vi "Open Device.vi"(8 "error in (no error)":errorcluster, 11 "Simulated Scope in":refnum<class "Simulated Scope.lvclass">) -> (0 "error out":errorcluster, 3 "Simulated Scope out":refnum<class "Simulated Scope.lvclass">)   [LabVIEW 2020, in "Simulated Scope.lvlib" / "Simulated Scope.lvclass"]
uses:
  Simulated Scope.lvclass
  Simulated Scope.lvclass/Simulated Scope.ctl
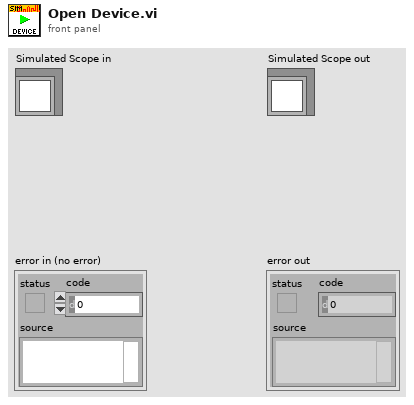
[diagram p1: front panel]
types:
  T1 = typedef "Simulated Scope.lvlib/Simulated Scope.lvclass/Ref Data.ctl" = cluster{"Sim Queue Name":string, "Waveform Queue":refnum<queue>}
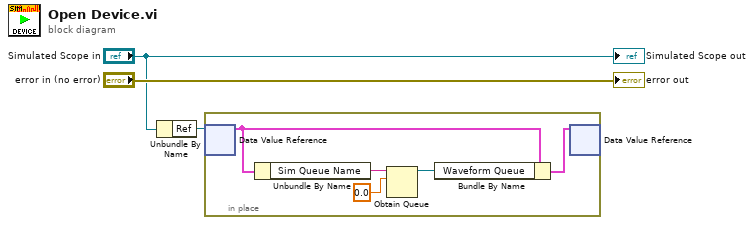
[diagram p0: block diagram]
diagram:
  n1 = Unbundle By Name("Simulated Scope in") -> ("Ref"=w3:refnum<data-value>)
  n2 = in-place {
    n3 = in-place-dvr #1(w3) -> (w6:T1)  [unwired: 1 out]
    n4 = Unbundle By Name(w6) -> ("Sim Queue Name"=w8:string)
    n5 = Obtain Queue(name (unnamed)=w8, element data type=0.0) -> (queue out=w5:refnum<queue>)  [unwired: 3 in, 2 out]
    n6 = Bundle By Name(cluster=w6, "Waveform Queue"=w5) -> (w4:T1)
    n7 = in-place-dvr #1(w4) -> ()  [unwired: 2 out]
  }
  "error out" <- "error in (no error)"
  "Simulated Scope out" <- "Simulated Scope in"
